vi "Init Actor Core.vi"(8 "error in (no error)":errorcluster, 11 "Measure Object in":refnum<class "LabActor.lvclass">) -> (0 "error out":errorcluster, 3 "Measure Object out":refnum<class "LabActor.lvclass">)   [LabVIEW 2024, in "LabActor.lvclass"]
uses:
  LabActor.lvclass
  <vilib>/Utility/miscctls.llb/LVRectTypeDef.ctl
  <vilib>/Utility/miscctls.llb/LVPointTypeDef.ctl
  Template Module/Template Module.lvclass/Template Module.ctl
  LabActor.lvclass/LabActor.ctl
  Template Module/Read Front Panel ref.vi
  Controllers/Application Controller/Application Controller.lvclass
panel:
  out "Origin":T1
  out "Front Panel Window:Panel Bounds":T2
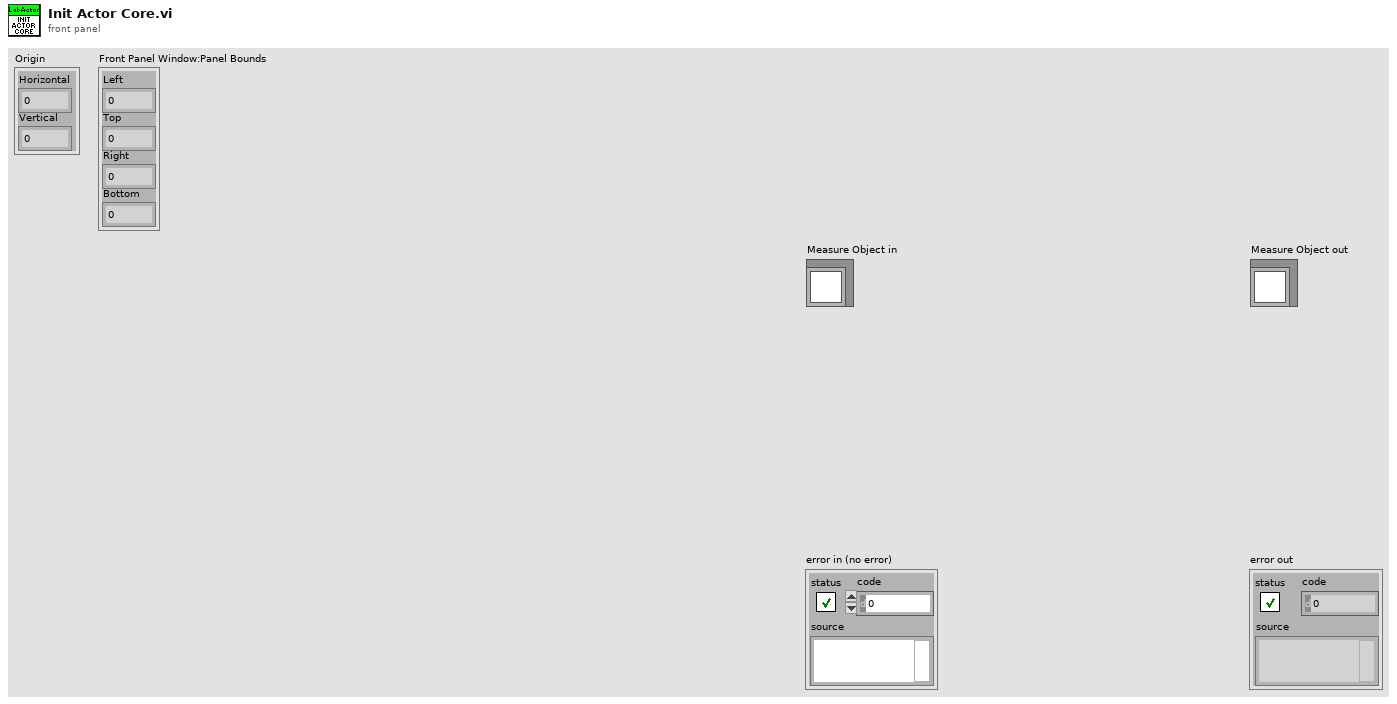
[diagram p1: front panel]
types:
  T1 = typedef "LVPointTypeDef.ctl" = cluster{"Horizontal":i16, "Vertical":i16}
  T2 = typedef "LVRectTypeDef.ctl" = cluster{"Left":i16, "Top":i16, "Right":i16, "Bottom":i16}
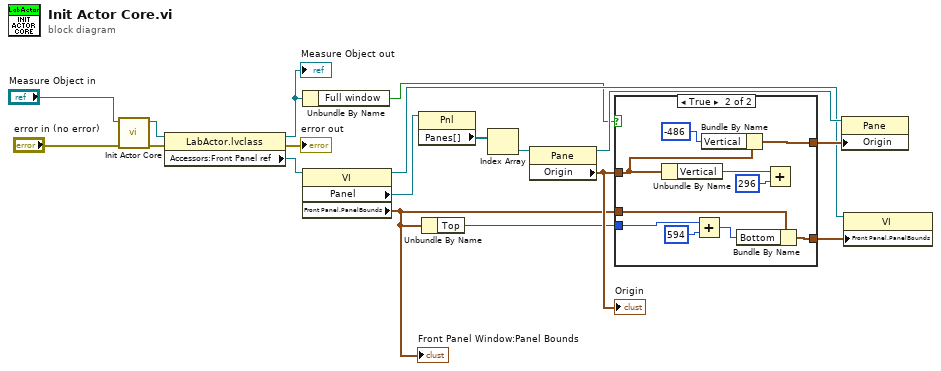
[diagram p0: block diagram]
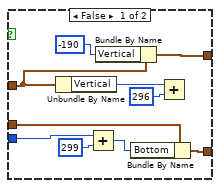
[diagram p2: hidden frame]
diagram:
  n1 = call-parent "Init Actor Core.vi"("error in (no error)"="error in (no error)", "Application Controller in"="Measure Object in") -> ("error out"=w18:errorcluster, "Application Controller out"=w14:refnum<class "LabActor.lvclass">)  [unwired: 8 in]
  n2 = property class="LabActor.lvclass"(reference=w14, error in=w18) -> (reference out=w12:refnum<class "LabActor.lvclass">, error out=→"error out":errorcluster, "Accessors:Front Panel ref"=w13:refnum<vi>)
  "Measure Object out" <- w12
  n3 = Unbundle By Name(w12) -> ("Full window"=w1:bool)
  n4 = property class="VI"(reference=w13) -> (reference out=w4:refnum<vi>, "Panel"=w11:refnum<vi>, "Front Panel.PanelBounds"=w2:T2)  [unwired: 1 in, 1 out]
  "Front Panel Window:Panel Bounds" <- w2
  n5 = property class="Pnl"(reference=w11) -> ("Panes[]"=w10:refnum<vi>[])  [unwired: 1 in, 2 out]
  n6 = Unbundle By Name(w2) -> ("Top"=w3:i16)
  n7 = Index Array(array=w10) -> (element=w9:refnum<vi>)  [unwired: 1 in]
  n8 = property class="Pane"(reference=w9) -> (reference out=w8:refnum<vi>, "Origin"=w7:T1)  [unwired: 1 in, 1 out]
  "Origin" <- w7
  n9 = case shown="True" w1 {
    tunnel: w7 -> [w27 w37]
    tunnel: [w26 w36] -> w6
    tunnel: [w24 w34] -> w5
    tunnel: w3 -> [w22 w32]
    tunnel: w2 -> [w19 w29]
    frame False {
      n10 = Unbundle By Name(w27) -> ("Vertical"=w28:i16)
      n11 = Add(x=w22, y=i16 299) -> (x+y=w20:i16)
      n12 = Bundle By Name(cluster=w27, "Vertical"=i16 -190) -> (w26:T1)
      n13 = Bundle By Name(cluster=w19, "Bottom"=w20) -> (w24:T2)
      n14 = Add(x=w28, y=i16 296) -> ()  [unwired: 1 out]
    }
    frame True {
      n15 = Unbundle By Name(w37) -> ("Vertical"=w38:i16)
      n16 = Add(x=w32, y=i16 594) -> (x+y=w30:i16)
      n17 = Bundle By Name(cluster=w37, "Vertical"=i16 -486) -> (w36:T1)
      n18 = Bundle By Name(cluster=w29, "Bottom"=w30) -> (w34:T2)
      n19 = Add(x=w38, y=i16 296) -> ()  [unwired: 1 out]
    }
  }
  n20 = property class="Pane"(reference=w8, "Origin"=w6) -> ()  [unwired: 1 in, 2 out]
  n21 = property class="VI"(reference=w4, "Front Panel.PanelBounds"=w5) -> ()  [unwired: 1 in, 2 out]
